vi "test Regex Matches Then Test Passes - Complex Regex.vi"(8 "error in (no error)":errorcluster, 11 "TestCase in":refnum<class "String Regex Test Case.lvclass">) -> (0 "error out":errorcluster, 3 "TestCase out":refnum<class "String Regex Test Case.lvclass">)   [LabVIEW 2015, in "String Regex Test Case.lvclass"]
uses:
  String Regex Test Case.lvclass
  <vilib>/addons/_JKI Toolkits/VI Tester/TestCase.llb/TestCase.lvclass
  VITAC.lvlib
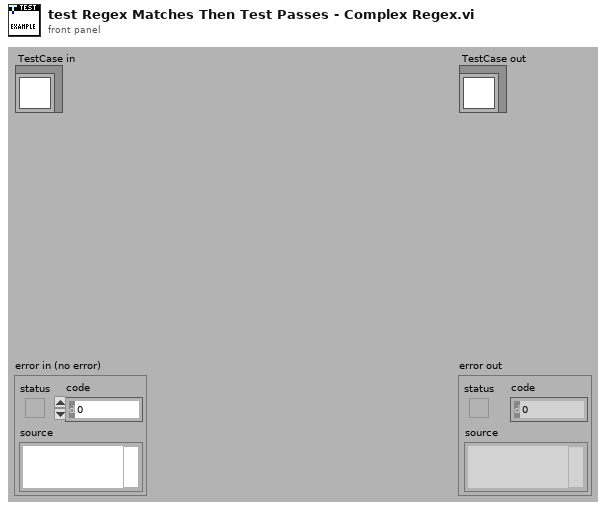
[diagram p1: front panel]
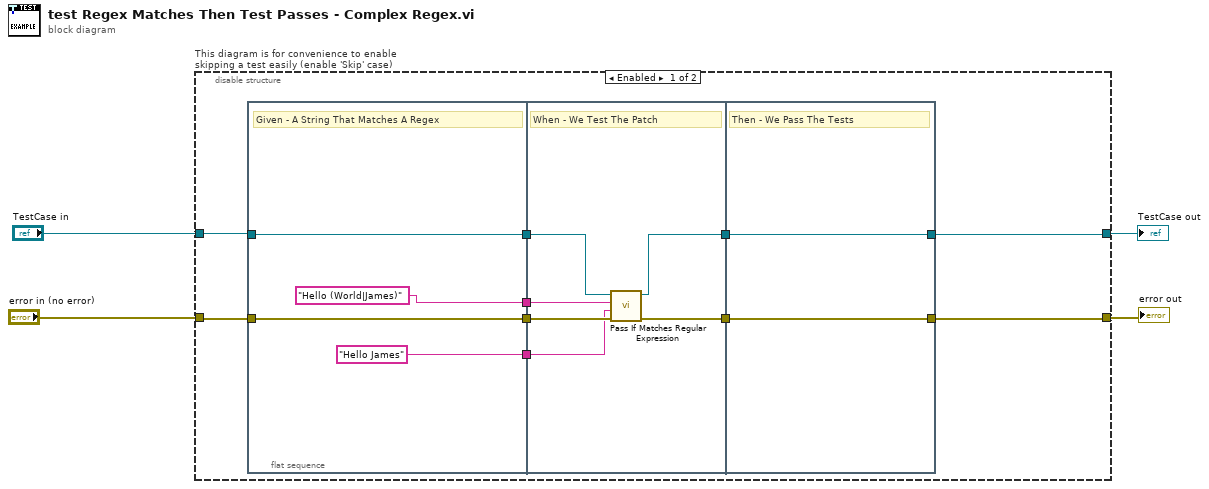
[diagram p0: block diagram]
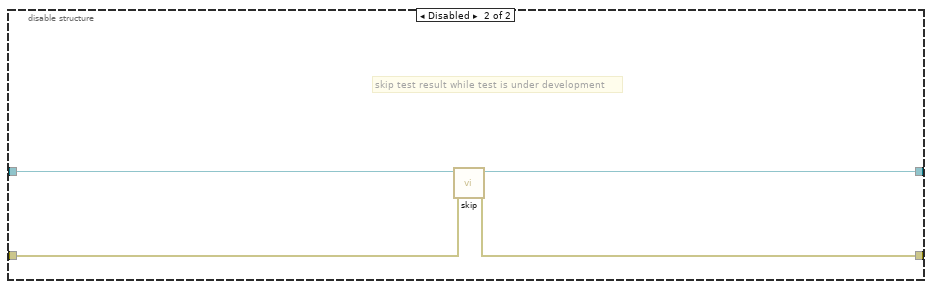
[diagram p2: hidden frame]
diagram:
  n1 = disable-structure "This diagram is for convenience to enable skipping a test easily (enable 'Skip' case)" shown="Enabled" {
    disable-tunnel: "TestCase in" -> [w10 w30]
    disable-tunnel: [w8 w28] -> w1
    disable-tunnel: [w7 w29] -> w3
    disable-tunnel: "error in (no error)" -> [w9 w27]
    frame Enabled {
      n2 = flat-sequence {
        tunnel: w9 -> [w17]
        tunnel: w10 -> [w18]
        tunnel: [w18] -> w14
        tunnel: [w17] -> w13
        tunnel: ["Hello James" ("actual")] -> w6
        tunnel: ["Hello (World|James)" ("actual")] -> w5
        tunnel: [w21] -> w12
        tunnel: [w23] -> w11
        tunnel: w14 -> [w22]
        tunnel: w13 -> [w24]
        tunnel: w6 -> [w20]
        tunnel: w5 -> [w19]
        tunnel: w12 -> [w26]
        tunnel: w11 -> [w25]
        tunnel: [w26] -> w8
        tunnel: [w25] -> w7
        frame #0 {
          # "Given - A String That Matches A Regex"
        }
        frame #1 {
          # "When - We Test The Patch"
          n3 = call "Pass If Matches Regular Expression.vi"("error in (no error)"=w24, "actual"=w20, "regular expression"=w19, "TestCase in"=w22) -> ("error out"=w23:errorcluster, "TestCase out"=w21:refnum<class "String Regex Test Case.lvclass">)  [unwired: 6 in]
        }
        frame #2 {
          # "Then - We Pass The Tests"
        }
      }
    }
    frame Disabled {
      # "skip test result while test is under development"
      n4 = call <vilib>:"skip.vi"("error in (no error)"=w27, "TestCase in"=w30) -> ("error out"=w29:errorcluster, "TestCase out"=w28:refnum<class "String Regex Test Case.lvclass">)  [unwired: 8 in]
    }
  }
  "error out" <- w3
  "TestCase out" <- w1
